vi "Stop Nested.vi"(10 "Final Code":i32, 11 "Actor API in":refnum<class "Actor API.lvclass">) -> (3 "Actor API out":refnum<class "Actor API.lvclass">)   [LabVIEW 2020, in "Artifex.lvlib" / "Actor API.lvclass"]
uses:
  Actor API.lvclass
  Priority Message Queue/Priority Message Queue.lvclass
  Priority.ctl
  Artifex.lvlib
  Stop Msg/Stop Msg.lvclass
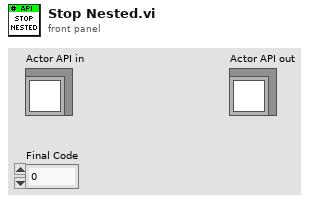
[diagram p1: front panel]
types:
  T1 = typedef "Artifex.lvlib/Priority.ctl" = enum16{"Low", "Normal", "High"}
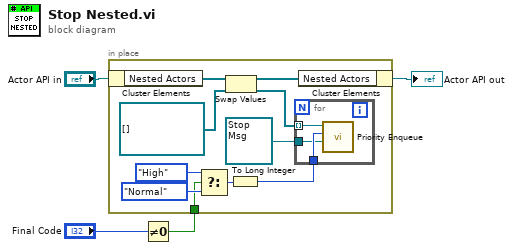
[diagram p0: block diagram]
diagram:
  n1 = Not Equal To 0?(x="Final Code") -> (x != 0?=w1:bool)
  n2 = in-place {
    in-place-border: w1 -> [w6]
    n3 = in-place-cluster #1("Actor API in") -> ("Nested Actors"=w14:refnum<class "Priority Message Queue.lvclass">[])
    n4 = Select(t=Priority."High" ("Priority"), s=w6, f=Priority."Normal" ("Priority")) -> (s? t:f=w8:T1)
    n5 = Swap Values(12:w14, 14:refnum<class "Priority Message Queue.lvclass">[] [] ("Nested Actors")) -> (1:w13:refnum<class "Priority Message Queue.lvclass">[], 3:w12:refnum<class "Priority Message Queue.lvclass">[])  [unwired: 1 in]
    n6 = To Long Integer(number=w8) -> (32bit integer=w7:i32)
    n7 = for {
      tunnel: w12 -> [w17] mode=indexing
      tunnel: w7 -> [w16]
      tunnel: refnum<class "Stop Msg.lvclass"> refnum ("Artifex.lvlib:Stop Msg.lvclass") -> [w15]
      n8 = call "Priority Enqueue.vi"("Message"=w15, "Priority"=w16, "Priority Message Queue in"=w17) -> ()  [unwired: 7 in, 2 out]
    }
    n9 = in-place-cluster #1("Nested Actors"=w13) -> (→"Actor API out":refnum<class "Actor API.lvclass">)
  }
